vi "Creating Points and Lines.vi"() -> ()   [LabVIEW 2016]
doc: "This VI demonstrates how to create points and lines in a 3D Picture using the Create Mesh with Attributes VI. It also demonstrates how to use the draw mode to generate points, lines, triangles, and polygons."
uses:
  <vilib>/Utility/miscctls.llb/LV3DPointTypeDef.ctl
  <vilib>/picture/3D Picture Control/Object/Create Object (drawable).vi
  <vilib>/picture/3D Picture Control/Object/Add Object (no reference).vi
  <vilib>/picture/3D Picture Control/Helpers/Set Light (no reference).vi
  <vilib>/picture/3D Picture Control/NI_3D Picture Control.lvlib
panel:
  in  "Stop":bool
  in  "Points":T1[](array[typedef])=[{"X"=1.0, "Y"=0.0, "Z"=0.0}, {"X"=0.0, "Y"=1.0, "Z"=0.0}, {"X"=0.0, "Y"=0.0, "Z"=1.0}, {"X"=0.0, "Y"=2.0, "Z"=1.0}]
  in  "Size":dbl(slide)=10.0 scale=0.0..10.0
  in  "Draw Mode":T2(ring)
  out "3D Picture":refnum<vi>(3d-picture)
  # "Overview: This VI demonstrates how to create points, lines, triangles, and polygons in a 3D Picture using the Create Mesh with Attributes VI.\nRequirements: LabVIEW Full Development System\nInstructions: \n1. Run the VI. \n2. Select the Draw Mode to specify how the points are rendered in the 3D Picture.\n3. Change the Size of the points and the location of the points in the Points array.\n4. Click Stop to stop the VI."
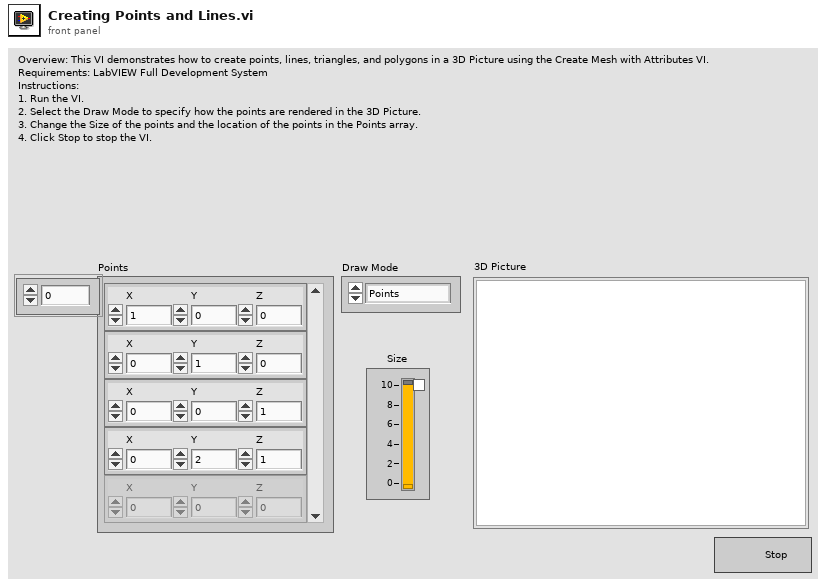
[diagram p1: front panel]
types:
  T1 = typedef "LV3DPointTypeDef.ctl" = cluster{"X":sgl, "Y":sgl, "Z":sgl}
  T2 = enum16{"Points", "Lines", "Line Strip", "Line Loop", "Triangles", "Triangle Strip", "Triangle Fan", "Quads", "Quad Strip", "Polygon"}
  T3 = enum16{"Inherit Value", "Points", "Wireframe", "Polygons"}
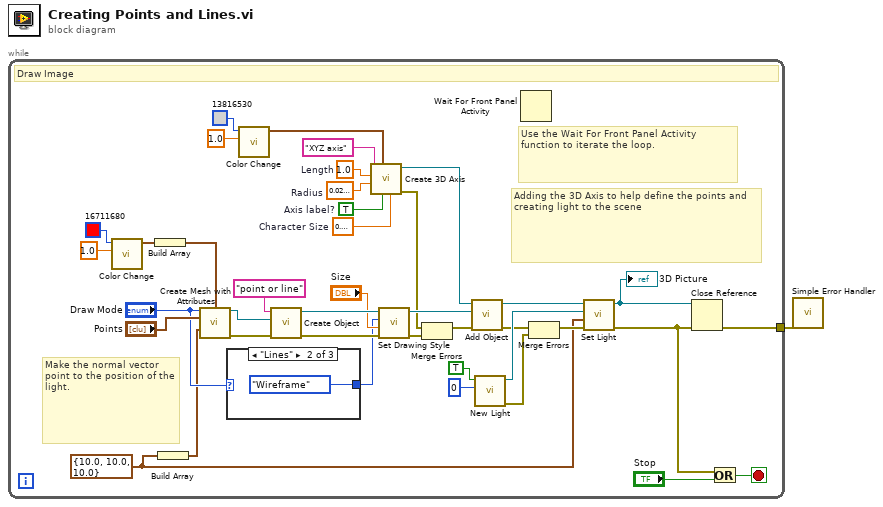
[diagram p0: block diagram]
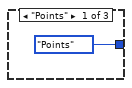
[diagram p2: hidden frame]
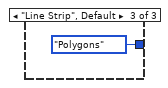
[diagram p3: hidden frame]
diagram:
  n1 = while {
    tunnel: [w2] -> w1
    stop <- w5 stop-if-true
    w9 = sgl 0.3  # Character Size
    w8 = T1 {"X"=10.0, "Y"=10.0, "Z"=10.0} ("Position")
    w28 = sgl 1.0  # Length
    w32 = sgl 0.03  # Radius
    w33 = TRUE  # Axis label?
    # "Use the Wait For Front Panel Activity function to iterate the loop."
    # "Adding the 3D Axis to help define the points and creating light to the scene"
    # "Make the normal vector point to the position of the light."
    # "Draw Image"
    n2 = call <vilib>:"Color Change.vi"("Alpha"=1.0, "Color"=u32 16711680) -> ("RGBA"=w37:cluster{"R":sgl, "G":sgl, "B":sgl, "A":sgl})  [unwired: 9 in]
    n3 = Build Array(w37) -> (w36:cluster{"R":sgl, "G":sgl, "B":sgl, "A":sgl}[])
    n4 = Build Array(w8) -> (w7:T1[])
    n5 = call <vilib>:"Create Mesh with Attributes.vi"("Draw Mode"="Draw Mode", "Color Array"=w36, "Vertex Array"="Points", "Normal Array"=w7) -> ("New Mesh Refnum"=w40:refnum<vi>, "error out"=w39:errorcluster)  [unwired: 10 in]
    n6 = case shown="\"Lines\"" "Draw Mode" {
      tunnel: [T3."Points" ("Mode") T3."Wireframe" ("Mode") T3."Polygons" ("Mode")] -> w10
      frame "Points" {
      }
      frame "Lines" {
      }
      frame "Line Strip", Default {
      }
    }
    n7 = call <vilib>:"Color Change.vi"("Alpha"=1.0, "Color"=u32 13816530) -> ("RGBA"=w29:cluster{"R":sgl, "G":sgl, "B":sgl, "A":sgl})  [unwired: 9 in]
    n8 = call-poly <vilib>:"Create Object.vi"("error in (no error)"=w39, "Geometry"=w40, "Name"="point or line") -> ("error out"=w21:errorcluster, "Scene:New Object"=w23:refnum<vi>)  [unwired: 7 in]
    n9 = call <vilib>:"Create 3D Axis.vi"("Character Size"=w9, "Axis label?"=w33, "Color"=w29, "Radius"=w32, "Length"=w28, "Name"="XYZ axis") -> ("error out"=w15:errorcluster, "New Object Refnum"=w16:refnum<vi>)  [unwired: 4 in]
    n10 = call <vilib>:"Set Drawing Style.vi"("error in (no error)"=w21, "Size"="Size", "Mode"=w10, "Scene Object In"=w23) -> ("error out"=w20:errorcluster, "Scene Object Out"=w22:refnum<vi>)  [unwired: 6 in]
    n11 = Merge Errors(w15, w20) -> (w18:errorcluster)
    n12 = call-poly <vilib>:"Add Object.vi"("error in (no error)"=w18, "New Object In"=w22, "Scene Object In"=w16) -> ("error out"=w14:errorcluster, "Scene Object Out"=w27:refnum<vi>)  [unwired: 7 in]
    n13 = call <vilib>:"New Light.vi"("Light Number"=0, "At Infinity"=TRUE) -> ("error out"=w12:errorcluster, "New Light Refnum"=w26:refnum<vi>)  [unwired: 8 in]
    n14 = Wait For Front Panel Activity() -> ()  [unwired: 3 in, 1 out]
    n15 = Merge Errors(w14, w12) -> (w13:errorcluster)
    n16 = call-poly <vilib>:"Set Light.vi"("error in (no error)"=w13, "Position"=w8, "Light Refnum In"=w26, "Scene Object In"=w27) -> ("error out"=w4:errorcluster, "Scene Object Out"=w3:refnum<vi>)  [unwired: 6 in]
    "3D Picture" <- w3
    n17 = Close Reference(reference=w3, error in (no error)=w4) -> (error out=w2:errorcluster)
    n18 = Or(x=w4, y="Stop") -> (x .or. y?=w5:bool)
  }
  n19 = call <vilib>:"Simple Error Handler.vi"("error in (no error)"=w1) -> ()  [unwired: 4 in, 5 out]
